vi "Save.vi"(0 "iUser Configuration Manager DVR":refnum<data-value>, 5 "Path":path, 11 "error in":errorcluster, 12 "Persistence":refnum<class "IPersist.lvclass">) -> (4 "dup iUser Configuration Manager DVR":refnum<data-value>, 15 "error out":errorcluster)   [LabVIEW 2017, in "User Configuration Manager.lvlib" / "By Ref.lvlib"]
uses:
  By Ref.lvlib
  iUser Configuration Manager/iUser Configuration Manager.lvclass
  <vilib>/gpm_packages/@cs/persistence/source/IPersist/IPersist.lvclass
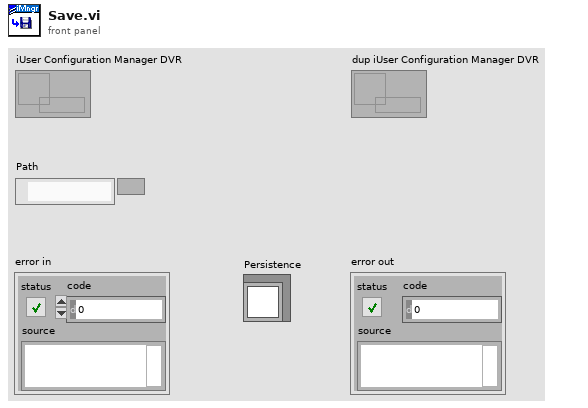
[diagram p1: front panel]
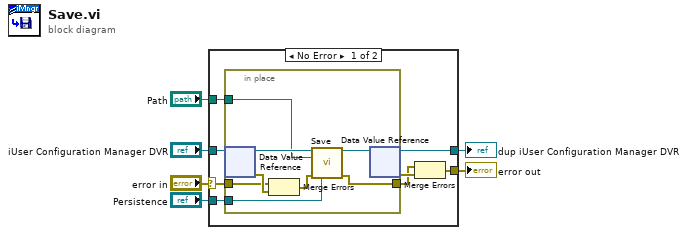
[diagram p0: block diagram]
diagram:
  n1 = case shown="No Error" "error in" {
    selector: "error in" -> [w12 w24]
    tunnel: "iUser Configuration Manager DVR" -> [w14 w23]
    tunnel: [w13 w24] -> w5
    tunnel: [w9 w23] -> w3
    tunnel: "Path" -> [w8 _]
    tunnel: "Persistence" -> [w7 _]
    frame No Error {
      n2 = in-place "IPES" {
        in-place-border: [w18] -> w10
        in-place-border: w12 -> [w21]
        in-place-border: w8 -> [w17]
        in-place-border: w7 -> [w15]
        n3 = in-place-dvr #1(w14) -> (w20:refnum<class "iUser Configuration Manager.lvclass">, w22:errorcluster)
        n4 = Merge Errors(w21, w22) -> (w16:errorcluster)
        n5 = call-dynamic "Save.vi"("iUser Configuration Manager in"=w20, "Path"=w17, "error in (no error)"=w16, "Persistence"=w15) -> ("iUser Configuration Manager out"=w19:refnum<class "iUser Configuration Manager.lvclass">, "error out"=w18:errorcluster)  [unwired: 10 in]
        n6 = in-place-dvr #1(w19) -> (w9:refnum<data-value>, w11:errorcluster)
      }
      n7 = Merge Errors(w10, w11) -> (w13:errorcluster)
    }
    frame Error {
    }
  }
  "error out" <- w5
  "dup iUser Configuration Manager DVR" <- w3
